vi "Configure.vi"(8 "error in (no error)":errorcluster, 11 "IMD in":refnum<class "IMD.lvclass">) -> (0 "error out":errorcluster, 3 "IMD out":refnum<class "IMD.lvclass">)   [LabVIEW 2020, in "IMD.lvclass"]
doc: "Configure the measurements paramaters to sweep.\nThis should be a pop up interface invoked by the configure test button on the main panel."
uses:
  IMD.lvclass
  Controls/Loop order.ctl
  IMD.lvclass/IMD.ctl
  Controls/Config info.ctl
panel:
  in  "IMD3":bool=TRUE caption="Third order IMD"
  in  "IMD2":bool caption="Second order IMD"
  in  "Stop level":dbl=999.0 caption="Stop if IMD higher than (dBm)"
  in  "Loop order":T1
  in  "Offset Frequency (MHz)":string="45"
  in  "Delta Power (dB)":string="0"
  in  "Power (dBm)":string="20:30/2"
  in  "Frequency (MHz)":string="900"
  in  "Un-even IMD Measurement":bool
  in  "OK Button":bool
  in  "Average On":bool
  in  "Number of Averages":dbl
  in  "VBW":dbl format="%#_6p"
  in  "RBW":dbl format="%#_6p"
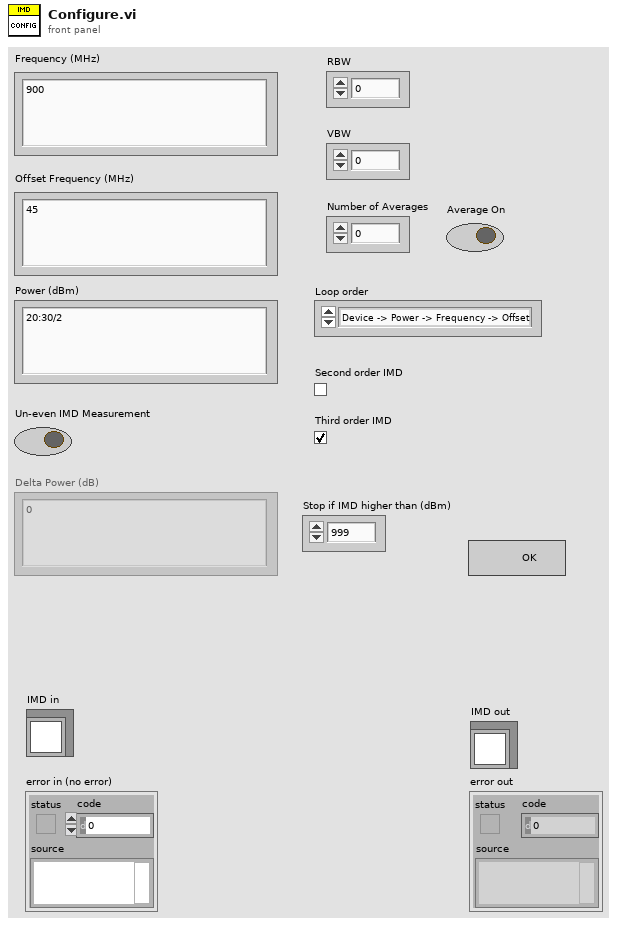
[diagram p1: front panel]
types:
  T1 = typedef "IMD.lvclass/Loop order.ctl" = enum16{"Device -> Power -> Frequency -> Offset", "Device -> Frequency -> Power -> Offset"}
  T2 = enum8{"Enabled", "Disabled", "Disabled and Grayed Out"}
  T3 = typedef "IMD.lvclass/Config info.ctl" = cluster{"RBW":dbl, "VBW ":dbl, "Number of Averages":dbl, "Average On":bool, "Frequency (MHz)":string, "Offset Frequency (MHz)":string, "Power (dBm)":string, "Delta Power (dB)":string, "Uneven IMD":bool, "Loop order":T1, "Stop level":dbl, "IMD2":bool, "IMD3":bool}
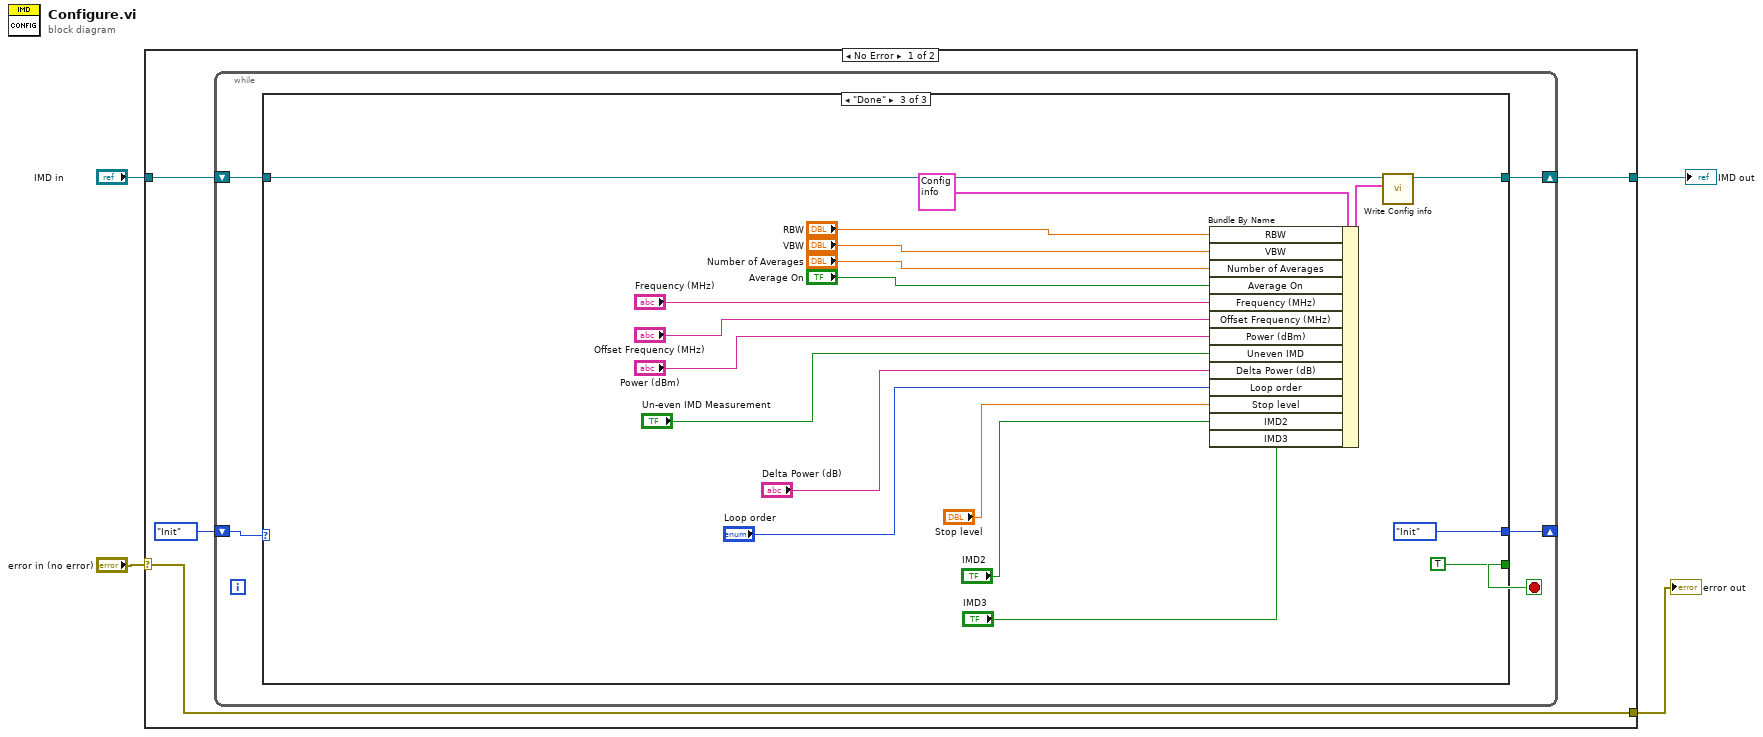
[diagram p0: block diagram]
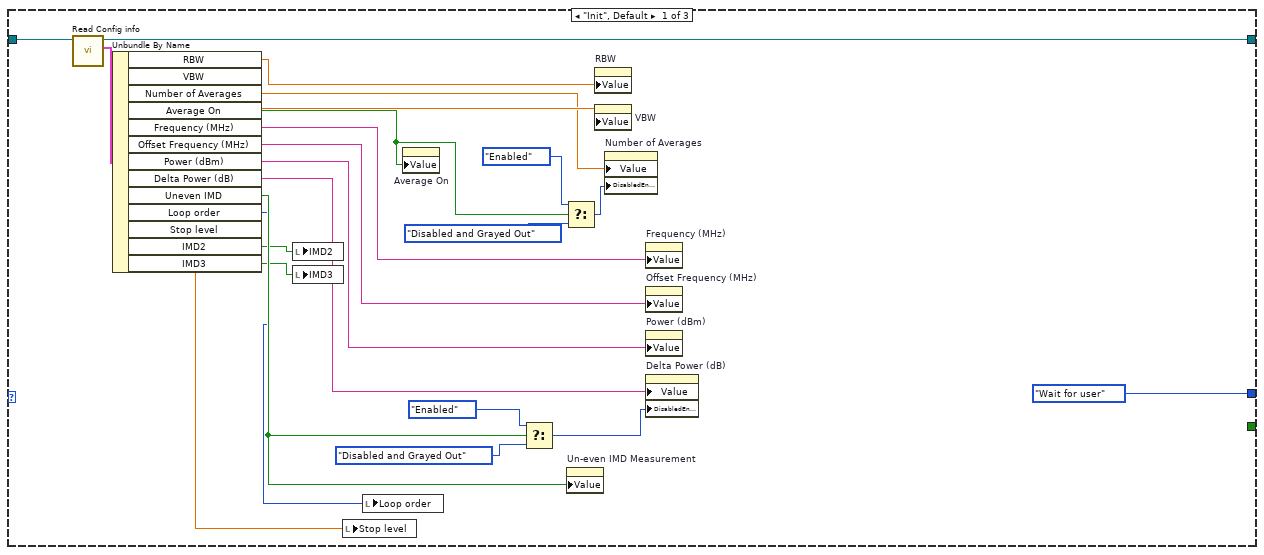
[diagram p2: hidden frame]
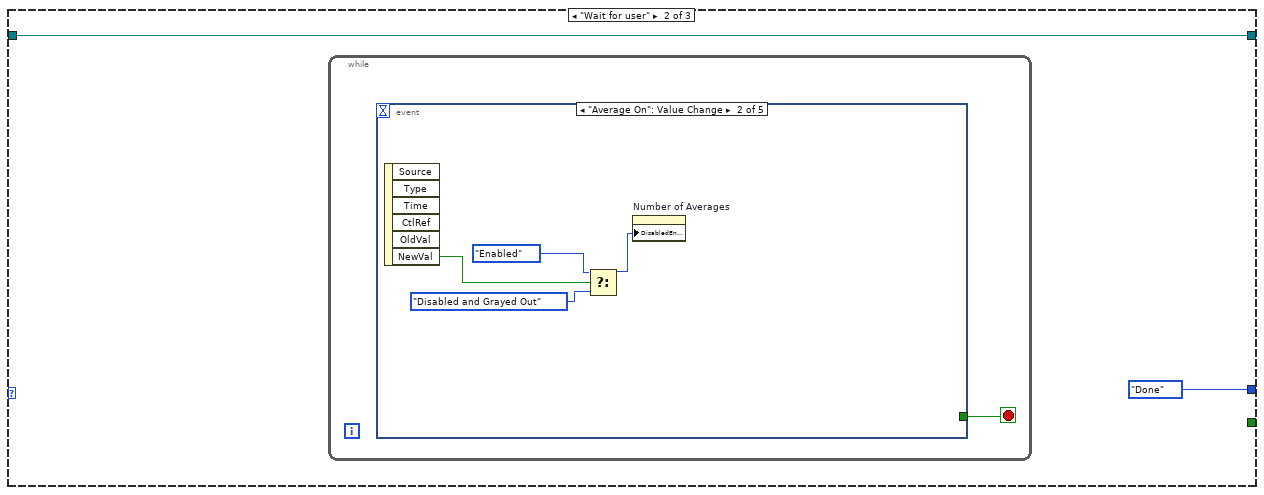
[diagram p3: hidden frame]
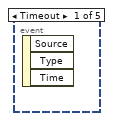
[diagram p4: hidden frame]
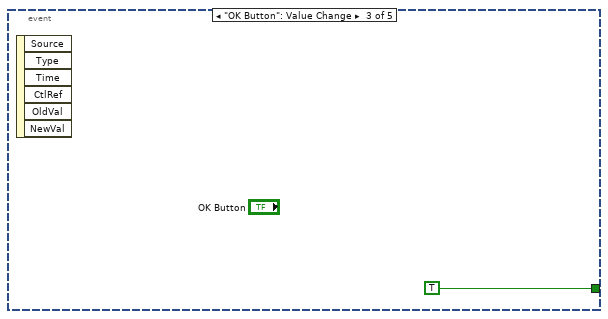
[diagram p5: hidden frame]
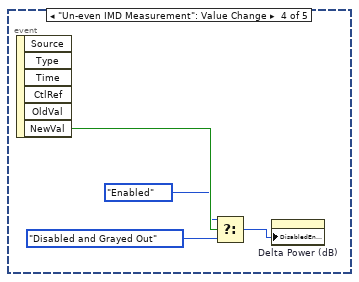
[diagram p6: hidden frame]
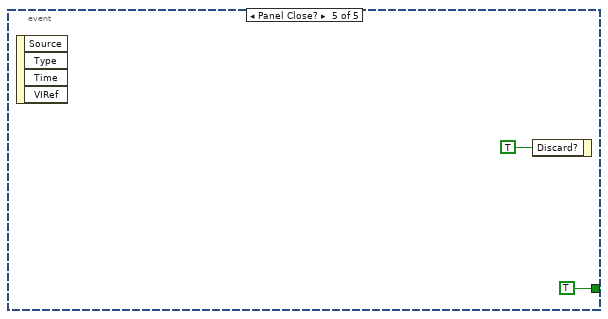
[diagram p7: hidden frame]
diagram:
  n1 = case shown="No Error" "error in (no error)" {
    selector: "error in (no error)" -> [w5 w70]
    tunnel: "IMD in" -> [w8 w71]
    tunnel: [w7 w71] -> w2
    tunnel: [w5 w70] -> w1
    frame No Error {
      n2 = while {
        shift-right: [w12] -> w7
        shift-left: w8 -> [w13]
        shift-right: [w10] -> _
        shift-left: enum16{"Init", "Wait for user", "Done"}."Init" -> [w11]
        stop <- w9 stop-if-true
        n3 = case shown="\"Done\"" w11 {
          tunnel: w13 -> [w36 w38 w66]
          tunnel: [w27 w38 w67] -> w12
          tunnel: [enum16{"Init", "Wait for user", "Done"}."Wait for user" enum16{"Init", "Wait for user", "Done"}."Done" enum16{"Init", "Wait for user", "Done"}."Init"] -> w10
          tunnel: [_ _ TRUE] -> w9
          frame "Init", Default {
            n4 = call "Read Config info.vi"("IMD in"=w36) -> ("Config info"=w35:T3, "IMD out"=w27:refnum<class "IMD.lvclass">)  [unwired: 9 in]
            n5 = Unbundle By Name(w35) -> ("RBW"=w34:dbl, "VBW"=w33:dbl, "Number of Averages"=w32:dbl, "Average On"=w28:bool, "Frequency (MHz)"=w20:string, "Offset Frequency (MHz)"=w19:string, "Power (dBm)"=w18:string, "Delta Power (dB)"=w22:string, "Uneven IMD"=w25:bool, "Loop order"=w16:T1, "Stop level"=w17:dbl, "IMD2"=w15:bool, "IMD3"=w14:bool)
            n6 = local write "IMD2"(w15) -> ()
            n7 = local write "IMD3"(w14) -> ()
            n8 = local write "Stop level"(w17) -> ()
            n9 = local write "Loop order"(w16) -> ()
            n10 = property on="Average On" class="Bool (strict)"("Value"=w28) -> ()  [unwired: 2 in, 2 out]
            n11 = Select(t=T2."Enabled" ("Disabled"), s=w25, f=T2."Disabled and Grayed Out") -> (s? t:f=w21:T2)
            n12 = Select(t=T2."Enabled" ("Disabled"), s=w28, f=T2."Disabled and Grayed Out") -> (s? t:f=w30:T2)
            n13 = property on="Un-even IMD Measurement" class="Bool (strict)"("Value"=w25) -> ()  [unwired: 2 in, 2 out]
            n14 = property on="RBW" class="DigNum (strict)"("Value"=w34) -> ()  [unwired: 2 in, 2 out]
            n15 = property on="VBW" class="DigNum (strict)"("Value"=w33) -> ()  [unwired: 2 in, 2 out]
            n16 = property on="Number of Averages" class="DigNum (strict)"("Value"=w32, "DisabledEnum"=w30) -> ()  [unwired: 2 in, 2 out]
            n17 = property on="Frequency (MHz)" class="Str"("Value"=w20) -> ()  [unwired: 2 in, 2 out]
            n18 = property on="Offset Frequency (MHz)" class="Str"("Value"=w19) -> ()  [unwired: 2 in, 2 out]
            n19 = property on="Power (dBm)" class="Str"("Value"=w18) -> ()  [unwired: 2 in, 2 out]
            n20 = property on="Delta Power (dB)" class="Str"("Value"=w22, "DisabledEnum"=w21) -> ()  [unwired: 2 in, 2 out]
          }
          frame "Wait for user" {
            n21 = while {
              stop <- w39 stop-if-true
              n22 = event shown="[1] \"Average On\": Value Change" {
                selector: _ -> [_ _ _ _ _]
                dyn-events: _ -> [_ _ _ _ _]
                timeout: _ -> [_ _ _ _ _]
                tunnel: [_ _ TRUE _ TRUE] -> w39
                event Timeout {
                  n23 = event-data() -> ()  [unwired: 1 in, 3 out]
                }
                event "Average On": Value Change {
                  n24 = event-data() -> ("NewVal"=w43:bool)  [unwired: 1 in, 5 out]
                  n25 = Select(t=T2."Enabled" ("Disabled"), s=w43, f=T2."Disabled and Grayed Out" ("Disabled")) -> (s? t:f=w42:T2)
                  n26 = property on="Number of Averages" class="DigNum (strict)"("DisabledEnum"=w42) -> ()  [unwired: 2 in, 2 out]
                }
                event "OK Button": Value Change {
                  n27 = event-data() -> ()  [unwired: 1 in, 6 out]
                }
                event "Un-even IMD Measurement": Value Change {
                  n28 = event-data() -> ("NewVal"=w48:bool)  [unwired: 1 in, 5 out]
                  n29 = Select(t=T2."Enabled" ("Disabled"), s=w48, f=T2."Disabled and Grayed Out") -> (s? t:f=w45:T2)
                  n30 = property on="Delta Power (dB)" class="Str"("DisabledEnum"=w45) -> ()  [unwired: 2 in, 2 out]
                }
                event Panel Close? {
                  n31 = event-data() -> ()  [unwired: 1 in, 4 out]
                  n32 = event-data("Discard?"=TRUE) -> ()  [unwired: 1 in, 1 out]
                }
              }
            }
          }
          frame "Done" {
            n33 = Bundle By Name(cluster=T3 {"RBW"=0.0, "VBW "=0.0, "Number of Averages"=0.0, "Average On"=FALSE, "Frequency (MHz)"="900", "Offset Frequency (MHz)"="45", "Power (dBm)"="20:30/2", "Delta Power (dB)"="20:30/2", "Uneven IMD"=FALSE, "Loop order"=enum."Device -> Power -> Frequency -> Offset", "Stop level"=999.0, "IMD2"=FALSE, "IMD3"=FALSE} ("Config info"), "RBW"="RBW", "VBW"="VBW", "Number of Averages"="Number of Averages", "Average On"="Average On", "Frequency (MHz)"="Frequency (MHz)", "Offset Frequency (MHz)"="Offset Frequency (MHz)", "Power (dBm)"="Power (dBm)", "Uneven IMD"="Un-even IMD Measurement", "Delta Power (dB)"="Delta Power (dB)", "Loop order"="Loop order", "Stop level"="Stop level", "IMD2"="IMD2", "IMD3"="IMD3") -> (w60:T3)
            n34 = call "Write Config info.vi"("Config info"=w60, "IMD in"=w66) -> ("IMD out"=w67:refnum<class "IMD.lvclass">)  [unwired: 9 in]
          }
        }
      }
    }
    frame Error {
    }
  }
  "error out" <- w1
  "IMD out" <- w2
